vi "Run_UTF.vi"(7 "LabVIEW Web Service Request":refnum<class "Web Request.lvclass">, 11 "JSON":string) -> (3 "Result":string)   [LabVIEW 2014]
uses:
  <vilib>/wsapi/Web Request.lvclass
  <vilib>/wsapi/NI_WebServices.lvlib
  Run UTF/Run UTF.lvclass
panel:
  out "error out":errorcluster
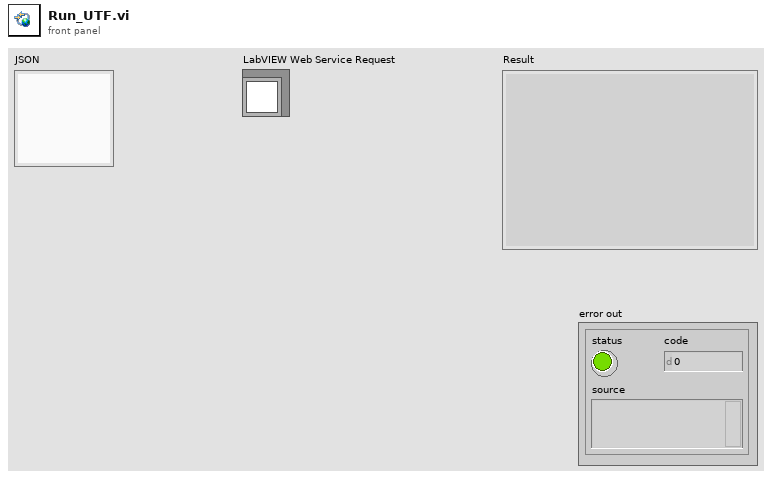
[diagram p1: front panel]
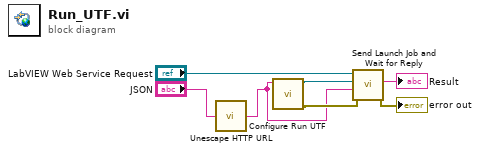
[diagram p0: block diagram]
diagram:
  n1 = call <vilib>:"Unescape HTTP URL.vi"("escaped string in"="JSON") -> ("unescaped string out"=w1:string)
  n2 = call "Configure Run UTF.vi"("JSON string"=w1) -> ("error out"=w3:errorcluster, "Run UTF.lvclass"=w2:refnum<class "Run UTF.lvclass">)  [unwired: 9 in]
  n3 = call "Send Launch Job and Wait for Reply.vi"("error in (no error)"=w3, "JSON"=w1, "Job"=w2, "Web Request in"="LabVIEW Web Service Request") -> ("error out"=→"error out":errorcluster, "Result String"=→"Result":string)  [unwired: 6 in]
